vi "Self Configure.vi"(8 "error in":errorcluster, 11 "34980A in":refnum<class "34980A.lvclass">) -> (0 "error out":errorcluster, 3 "34980A out":refnum<class "34980A.lvclass">)   [LabVIEW 2019, in "34980A.lvlib" / "34980A.lvclass"]
uses:
  Library/34980A.lvclass
  Custom Controls/Configuration Keys.ctl
  Library/34980A.lvclass/34980A.ctl
  builds/Instruments/MLTFNC.lvlibp/Library/MLTFNC.lvclass
  builds/Tools/Config.lvlibp/Config.lvclass
  C:/Users/Public/Documents/Development/builds/Tools/Config.lvlibp/Config.lvclass
panel:
  in  "Configuration Keys":T1
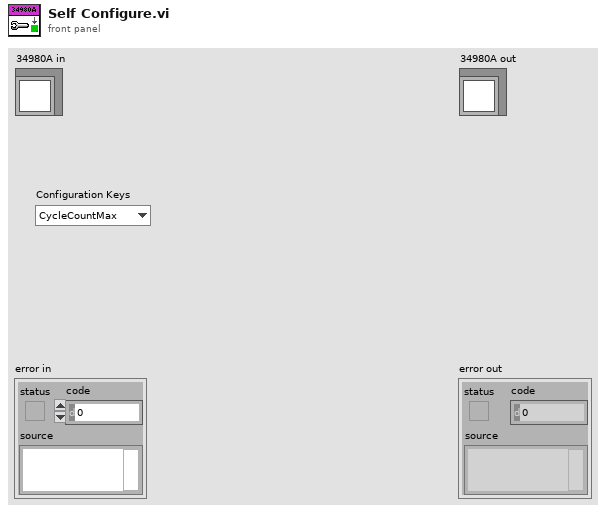
[diagram p1: front panel]
types:
  T1 = typedef "34980A.lvlib/34980A.lvclass/Configuration Keys.ctl" = enum16{"CycleCountMax"}
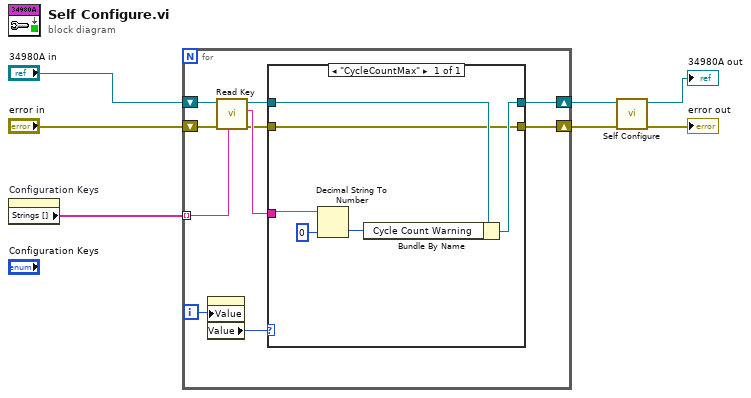
[diagram p0: block diagram]
diagram:
  n1 = property on="Configuration Keys" class="Enum (strict)"() -> ("Strings []"=w5:string[])  [unwired: 2 in, 2 out]
  n2 = for {
    tunnel: w5 -> [w13] mode=indexing
    shift-right: [w11] -> w3
    shift-left: "34980A in" -> [w15]
    shift-right: [w8] -> w1
    shift-left: "error in" -> [w10]
    i -> [w17]
    n3 = property on="Configuration Keys" class="Enum (strict)"("Value"=w17) -> ("Value"=w16:T1)  [unwired: 2 in, 2 out]
    n4 = call "Read Key.vi"("Key Name"=w13, "error in"=w10, "Config in"=w15) -> ("error out"=w9:errorcluster, "Key Value"=w12:string, "Config out"=w14:refnum<class "34980A.lvclass">)  [unwired: 6 in]
    n5 = case shown="\"CycleCountMax\"" w16 {
      tunnel: w14 -> [w22]
      tunnel: w12 -> [w23]
      tunnel: [w21] -> w11
      tunnel: w9 -> [w18]
      tunnel: [w18] -> w8
      frame "CycleCountMax" {
        n6 = Decimal String To Number(string=w23, default (0L)=u32 0 ("default (0 I32)")) -> (number=w20:u32)  [unwired: 1 in, 1 out]
        n7 = Bundle By Name(cluster=w22, "Cycle Count Warning"=w20) -> (w21:refnum<class "34980A.lvclass">)
      }
    }
  }
  n8 = call-parent "Self Configure.vi"("error in"=w1, "MLTFNC in"=w3) -> ("error out"=→"error out":errorcluster, "MLTFNC out"=→"34980A out":refnum<class "34980A.lvclass">)  [unwired: 8 in]
